vi "ContRunAuxPulse.vi"(6 "camera":bool, 7 "Aux pulse in":T2, 8 "error in (no error)":errorcluster, 10 "image size":cluster{"xpixels":i32, "ypixels":i32}) -> (0 "error out":errorcluster, 3 "READOUT":T1)   [LabVIEW 2019]
uses:
  PulseControl.ctl
  Compiler/Params.ctl
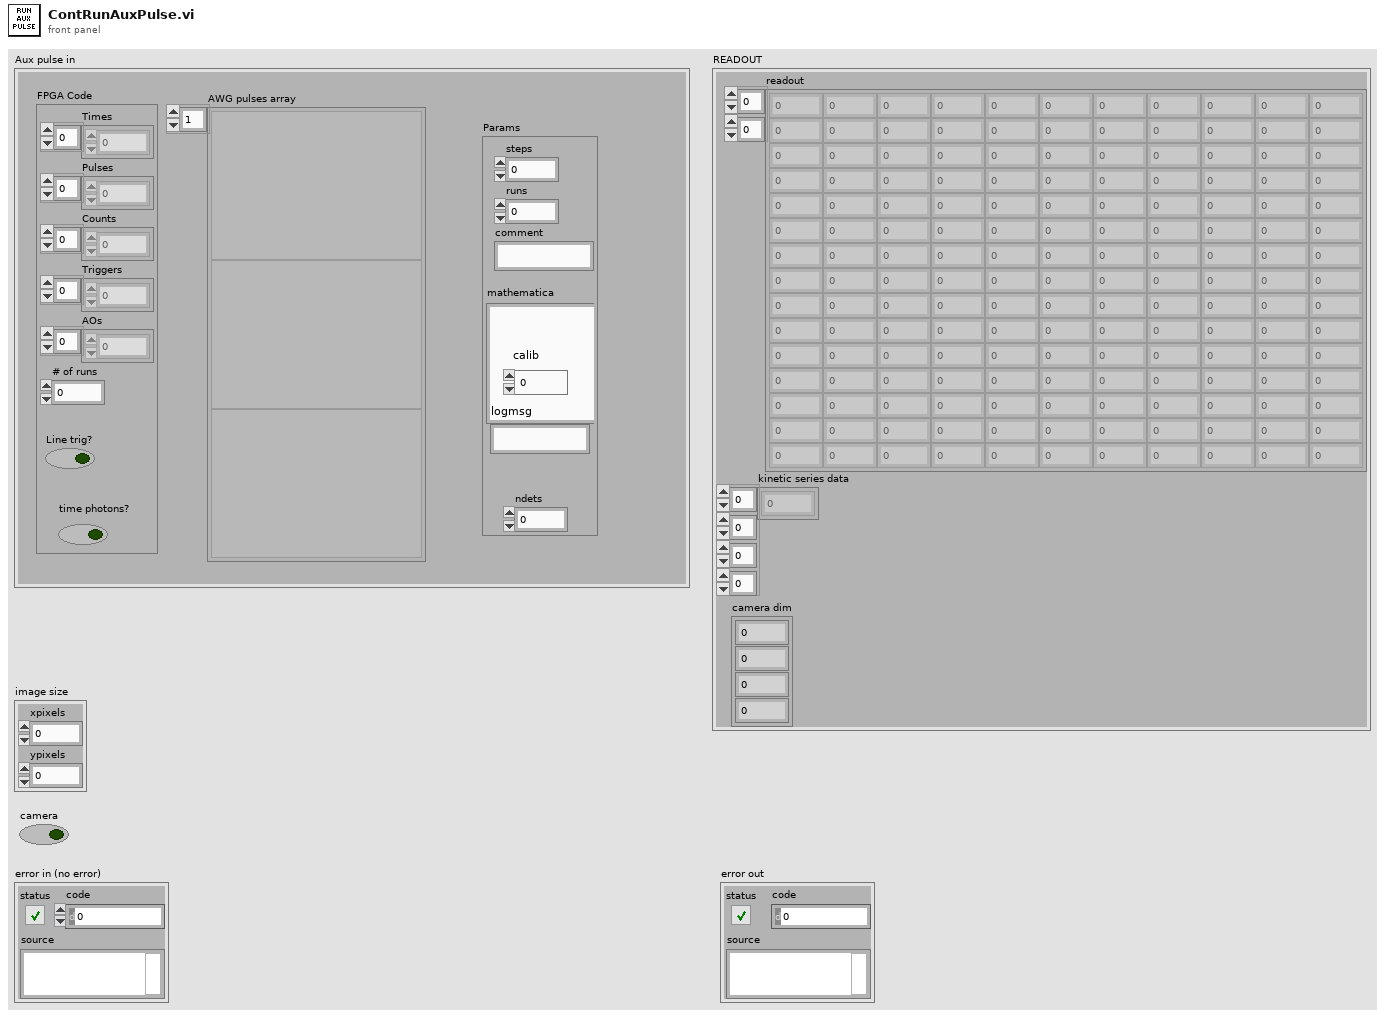
[diagram p1: front panel]
types:
  T1 = cluster{"readout":u32[][], "kinetic series data":i32[][][][], "camera dim":cluster{i32, i32, i32, i32}}
  T2 = typedef "PulseControl.ctl" = cluster{"FPGA Code":cluster{"Times":u32[], "Pulses":u64[], "Counts":u8[], "Triggers":u8[], "AOs":u8[], "# of runs":i32, "Line trig?":bool, "time photons?":bool}, "AWG pulses array":variant[], "Params":T3}
  T3 = typedef "Params.ctl" = cluster{"steps":i16, "runs":i16, "comment":string, "mathematica":string, "calib":i8, "logmsg":string, "ndets":i16}
  T4 = cluster{"Times":u32[], "Pulses":u64[], "Counts":u8[], "Triggers":u8[], "AOs":u8[], "# of runs":i32, "Line trig?":bool, "time photons?":bool}
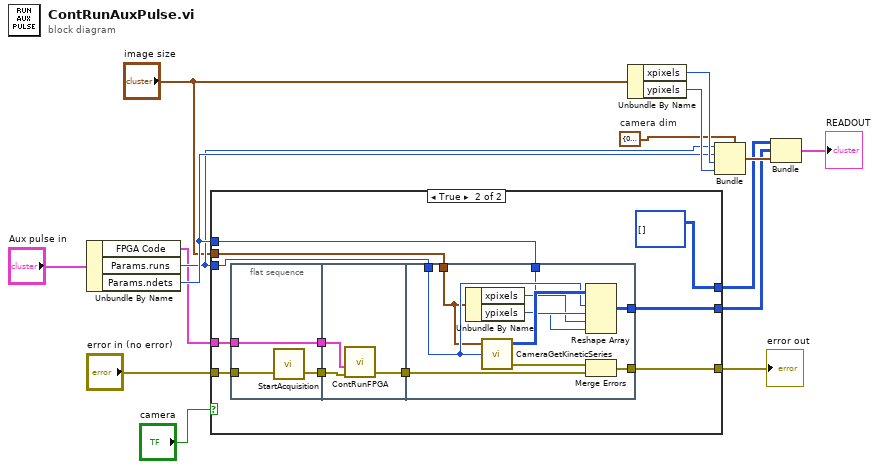
[diagram p0: block diagram]
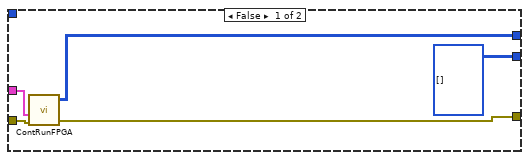
[diagram p2: hidden frame]
diagram:
  w5 = cluster{i32, i32, i32, i32} {0, 0, 0, 0}  # camera dim
  n1 = Unbundle By Name("Aux pulse in") -> ("FPGA Code"=w2:T4, "Params.runs"=w7:i16, "Params.ndets"=w8:i16)
  n2 = case shown="True" "camera" {
    tunnel: w2 -> [w20 w31]
    tunnel: [w17 u32[][] [] ("readout")] -> w3
    tunnel: "error in (no error)" -> [w19 w30]
    tunnel: [w18 w29] -> w15
    tunnel: w7 -> [_ w25]
    tunnel: w8 -> [_ w24]
    tunnel: [i32[][][][] [] ("kinetic series data") w23] -> w4
    tunnel: "image size" -> [_ w21]
    frame False {
      n3 = call "ContRunFPGA.vi"("error in"=w19, "Cluster"=w20) -> ("error out"=w18:errorcluster, "readout"=w17:i16[][])  [unwired: 2 in, 1 out]
    }
    frame True {
      n4 = flat-sequence {
        tunnel: w30 -> [w33]
        tunnel: w31 -> [w34]
        tunnel: [w34] -> w28
        tunnel: [w32] -> w27
        tunnel: w28 -> [w37]
        tunnel: w27 -> [w36]
        tunnel: [w35] -> w26
        tunnel: [w45] -> w29
        tunnel: w26 -> [w46]
        tunnel: w25 -> [w43]
        tunnel: w24 -> [w42]
        tunnel: [w39] -> w23
        tunnel: w21 -> [w38]
        frame #0 {
          n5 = call <userlib>:"StartAcquisition.vi"("error in (no error)"=w33) -> ("error out"=w32:errorcluster)  [unwired: 1 in, 1 out]
        }
        frame #1 {
          n6 = call "ContRunFPGA.vi"("error in"=w36, "Cluster"=w37) -> ("error out"=w35:errorcluster)  [unwired: 2 in, 2 out]
        }
        frame #2 {
          n7 = Unbundle By Name(w38) -> ("xpixels"=w41:i32, "ypixels"=w40:i32)
          n8 = call "CameraGetKineticSeries.vi"("# of kinetics"=w43, "image size"=w38) -> ("error out"=w47:errorcluster, "kinetic series data"=w44:i32[][][])  [unwired: 2 in]
          n9 = Reshape Array(w44, w43, w42, w41, w40) -> (w39:i32[][][][])
          n10 = Merge Errors(w47, w46) -> (w45:errorcluster)
        }
      }
    }
  }
  "error out" <- w15
  n11 = Unbundle By Name("image size") -> ("xpixels"=w9:i32, "ypixels"=w10:i32)
  n12 = Bundle(cluster=w5, w7, w8, w9, w10) -> (w6:cluster{i32, i32, i32, i32})
  n13 = Bundle("readout"=w3, "kinetic series data"=w4, "camera dim"=w6) -> (→"READOUT":T1)  [unwired: 1 in]
